vi "运维调试_采配水GD.vi"() -> ()   [LabVIEW 2016, in "PLC.lvlib"]
uses:
  PLC.lvlib
  control/switch.ctl
  <vilib>/Plasmionique/MB Master/MB_Master/MB_Master.lvclass
  <vilib>/Utility/miscctls.llb/LVPointTypeDef.ctl
  <vilib>/Plasmionique/MB Master/MB_Master_Serial/MB_Master_Serial.lvclass
  E:/Program Files (x86)/National Instruments/LabVIEW 2016/vi.lib/Plasmionique/MB Master/MB_Master/MB_Master.lvclass
  <vilib>/Plasmionique/MB Master/MB_Master_TCP/MB_Master_TCP.lvclass
  <vilib>/Plasmionique/MB Master/MB Master.lvlib
panel:
  in  "选项卡控件":enum32{"流程图", "控制面板"}(tab)
  in  "泵2进样阀":T1
  in  "泵1进样阀":T1
  in  "除藻泵阀":T2
  in  "自来水出水阀V7":T2
  in  "空压机阀":T3
  in  "增压泵M3":T4
  in  "空压机":T5
  in  "除藻泵M5":T6
  in  "泵1反冲洗阀V10":T2
  in  "泵2反冲洗阀V11":T2
  out "水流开关X2":T7
  in  "手动调节阀3":T8
  in  "采水泵M2":T9
  in  "采水泵M1":T9
  in  "氨氮水样池排液阀V15":T1
  in  "过滤反冲洗阀V14":T10
  in  "过滤进样阀V12":T11
  in  "配水泵M4":T3
  in  "过滤回流阀V13":T12
  in  "手动调节阀2":T13
  in  "压力开关":T14
  in  "手动调节阀":T8
  in  "流通池排液阀V4":T1
  in  "沉淀池排液阀V5":T1
  out "流通池液位开关X0":T15
  in  "沉淀池反冲洗阀-V9":T16
  in  "流通池反冲洗阀-V8":T16
  out "沉淀池液位开关X1":T15
  in  "M1":T17
  in  "M2":T17
  in  "V8":T17
  in  "V9":T17
  in  "V5":T17
  in  "V4":T17
  in  "V6":T17
  in  "V7":T17
  in  "V1":T17
  in  "V2":T17
  in  "V10":T17
  in  "V11":T17
  in  "M3":T17
  out "泵1进样阀计时":dbl
  out "泵2进样阀计时":dbl
  out "流通池反冲洗阀计时":dbl
  out "沉淀池反冲洗阀计时":dbl
  out "沉淀池排液阀计时":dbl
  out "流通池排液阀计时":dbl
  out "进气阀计时":dbl
  out "自来水出水阀计时":dbl
  out "泵1反冲洗阀计时":dbl
  out "泵2反冲洗阀计时":dbl
  out "M1工作计时":dbl
  out "M2工作计时":dbl
  out "增压泵计时":dbl
  in  "V3-G":T17
  in  "V3-R":T17
  out "流通池进样阀计时":dbl
  out "沉淀池进样阀计时":dbl
  in  "V13-R":T17
  in  "V14-G":T17
  in  "V12":T17
  in  "V13-G":T17
  in  "V14-R":T17
  out "过滤进样阀计时":dbl
  out "过滤回流阀计时":dbl
  out "过滤废水阀计时":dbl
  out "过滤反冲洗阀计时":dbl
  out "过滤出水阀计时":dbl
  in  "V15":T17
  in  "M4":T17
  out "氨氮水样池排液阀计时":dbl
  out "配水泵计时":dbl
  in  "63μm反冲洗阀":T17
  out "63μm反冲洗阀计时":dbl
  in  "除藻_M5":T17
  out "除藻计时":dbl
  in  "R124":u16(ring) caption="除藻工作模式" items=["手动", "自动"]
  out "R125":i16 caption="除藻时间"
  in  "连接设置":bool
  out "供水压力":sgl format="%#.4f"
  in  "63μm反冲洗阀启用":bool caption="63μm反冲洗阀"
  out "过滤压力":sgl format="%#.4f"
  in  "三级过滤系统":bool
  out "X8":bool caption="氨氮水样池液位开关_SL3"
  out "R122":i16 caption="氨氮水样池润洗时间"
  out "R123":i16 caption="过滤装置清洗时间"
  out "R121":i16 caption="过滤装置润洗时间"
  out "R120":i16 caption="加标回收配水时间"
  out "R116":i16 caption="储水时间设定"
  out "R115":i16 caption="清洗频次设定"
  out "R114":i16 caption="排液时间"
  out "R113":i16 caption="沉淀池清洗时间"
  out "R112":i16 caption="流通池清洗时间"
  out "R111":i16 caption="吹气时间"
  out "R110":i16 caption="外部管路清洗时间"
  out "R109":i16 caption="配水时间"
  out "R108":i16 caption="沉淀时间"
  out "R107":i16 caption="液位开关报警时间"
  out "R106":i16 caption="进样超时时间"
  out "R105":i16 caption="沉淀池润洗时间"
  out "R104":i16 caption="流通池润洗时间"
  out "状态":u16[](array[numeric])
  in  "更新程序":bool
  out "清洗次数":u16
  out "当前启动泵号":enum16{"1号泵", "2号泵"}(ring)
  in  "R117":u16(ring) caption="水箱储水水体" items=["自来水", "水样"]
  out "X2":bool caption="进样水流开关_JY"
  out "采配水版本号":string
  out "通讯故障":bool
  in  "R102":u16(ring) caption="采水泵工作模式" items=["泵1单泵单管路", "泵2单泵单管路", "双泵双管路"]
  out "X7":bool caption="烟雾报警_YW"
  out "X6":bool caption="泵2过载报警_KM2"
  out "X5":bool caption="泵1过载报警_KM1"
  out "X4":bool caption="外部电源断电报警_DD1"
  out "X3":bool caption="水浸报警_SJ"
  out "X1":bool caption="沉淀池液位开关_YE2"
  out "X0":bool caption="流通池液位开关_YE1"
  out "集成报警信息":string
  out "R2":i16
  out "R1":i16
  out "多列列表框":i32(listbox)
  in  "返回":bool
  in  "参数设置":bool
  in  "单步启动":bool
  in  "启动":bool
  in  "停止":bool
  # "S"
  # "S"
  # "S"
  # "S"
  # "S"
  # "S"
  # "S"
  # "S"
  # "S"
  # "S"
  # "S"
  # "S"
  # "S"
  # "S"
  # "次"
  # "S"
  # "S"
  # "S"
  # "供水压力："
  # "Mpa"
  # "过滤压力："
  # "Mpa"
  # "单步计时："
  # "s"
  # "流程计时："
  # "s"
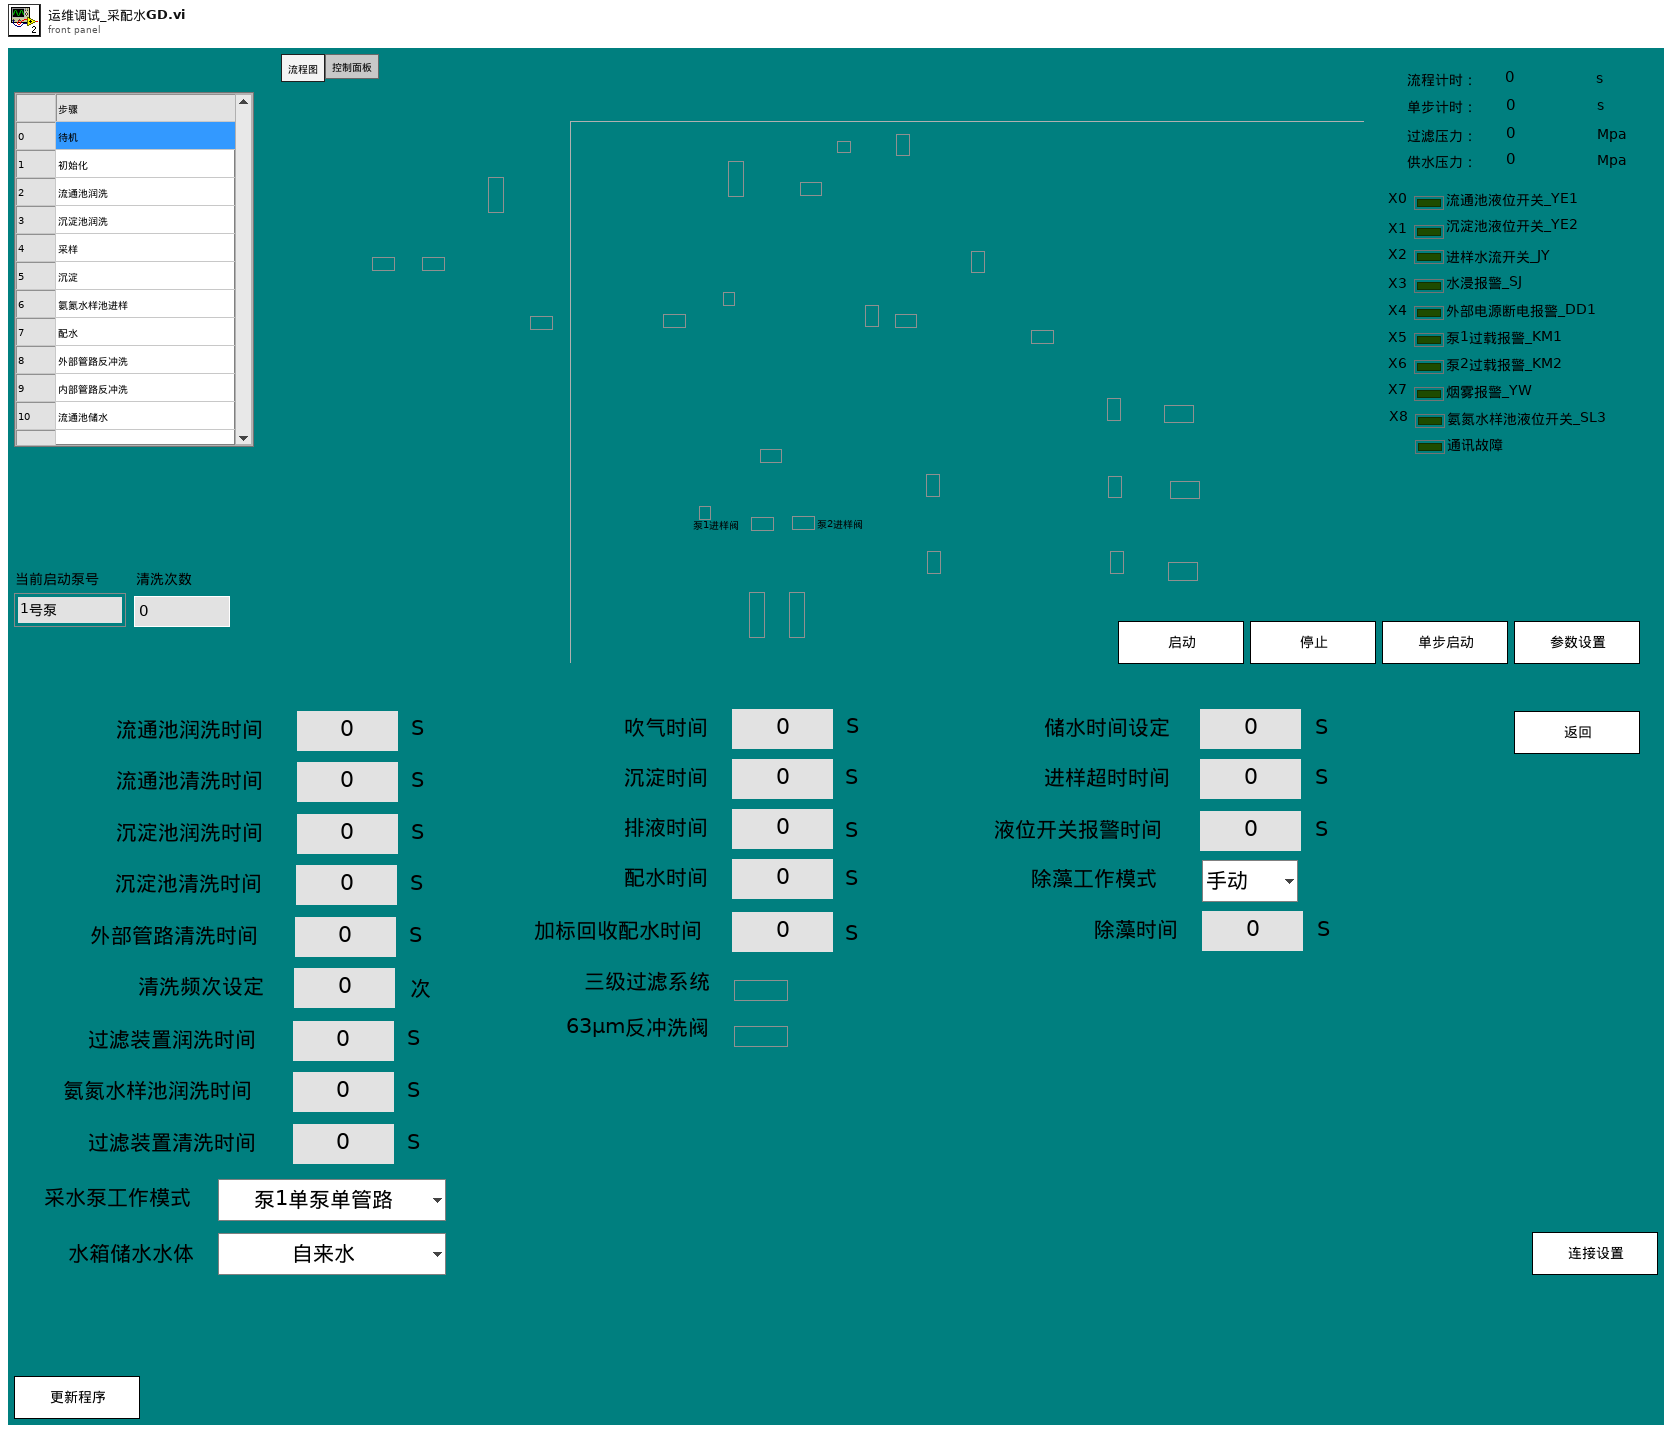
[diagram p1: front panel]
types:
  T1 = typedef "排液阀.ctl" = bool
  T2 = typedef "过滤进样阀.ctl" = bool
  T3 = typedef "电磁阀.ctl" = bool
  T4 = typedef "增压泵.ctl" = bool
  T5 = typedef "空压机.ctl" = bool
  T6 = typedef "除藻泵.ctl" = bool
  T7 = typedef "水流开关.ctl" = bool
  T8 = typedef "手动调节阀.ctl" = bool
  T9 = typedef "采水泵.ctl" = bool
  T10 = typedef "过滤出水阀.ctl" = bool
  T11 = typedef "过滤进样阀左.ctl" = bool
  T12 = typedef "三通电动球阀.ctl" = bool
  T13 = typedef "手动调节阀2.ctl" = bool
  T14 = typedef "压力开关.ctl" = bool
  T15 = typedef "浮子液位开关.ctl" = bool
  T16 = typedef "反冲洗阀.ctl" = bool
  T17 = typedef "PLC.lvlib/switch.ctl" = bool
  T18 = typedef "参数.ctl" = cluster{"测试模式":enum16{"水样测试", "平行样测试", "集成干预测试", "加标回收"}, "参数启用":T19}
  T19 = typedef "启动参数.ctl" = cluster{"氨氮":bool, "总磷":bool, "总氮":bool, "多参数":bool, "CODmn":bool, "CODCr":bool, "氟化物":bool, "超标留样":bool, "重金属":bool, "挥发酚":bool}
  T20 = cluster{"R100":i16, "R101":i16, "R102":i16, "R103":i16, "R104":i16, "R105":i16, "R106":i16, "R107":i16, "R108":i16, "R109":i16, "R110":i16, "R111":i16, "R112":i16, "R113":i16, "R114":i16, "R115":i16, "R116":i16, "R117":i16, "R118":i16, "R119":i16, "R120":i16, "R121":i16, "R122":i16, "R123":i16, "R124":i16, "R125":i16, "R126":i16, "R127":i16, "R128":i16, "R129":i16, "R130":i16, "R131":i16, "R132":i16, "R133":i16, "R134":i16, "R135":i16, "R136":i16}
  T21 = typedef "LVPointTypeDef.ctl" = cluster{"Horizontal":i16, "Vertical":i16}
  T22 = typedef "采配水类型.ctl" = enum16{"V1", "V2", "V3", "V4", "室内V1", "室内V2", "固定站V1", "固定站V2", "浮船V1", "浮船V2", "养殖渭水"}
  T23 = cluster{"R0":i16, "R1":i16, "R2":i16, "R3":i16, "R4":i16, "R5":i16, "R6":i16, "R7":i16, "R8":i16, "R9":i16, "R10":i16, "R11":i16, "R12":i16, "R13":i16, "R14":i16, "R15":i16, "R16":i16, "R17":i16, "R18":i16, "R19":i16, "R20":i16, "R21":i16, "R22":i16, "R23":i16, "R24":i16, "R25":i16, "R26":i16, "R27":i16, "R28":i16, "R29":i16, "R30":i16, "R31":i16, "R32":i16, "R33":i16, "R34":i16, "R35":i16, "R36":i16, "R37":i16, "R38":i16, "R39":i16, "R40":i16, "R41":i16, "R42":i16, "R43":i16, "R44":i16, "R45":i16, "R46":i16, "R47":i16, "R48":i16, "R49":i16, "R50":i16, "R51":i16, "R52":i16, "R53":i16, "R54":i16, "R55":i16, "R56":i16, "R57":i16, "R58":i16, "R59":i16, "R60":i16, "R61":i16, "R62":i16, "R63":i16, "R64":i16, "R65":i16, "R66":i16, "R67":i16, "R68":i16, "R69":i16, "R70":i16, "R71":i16, "R72":i16, "R73":i16, "R74":i16, "R75":i16, "R76":i16, "R77":i16, "R78":i16, "R79":i16}
  T24 = cluster{"seconds since 1Jan1904":timestamp, "table输入":string, string, "table输入":string}
  T25 = cluster{"命令":string, cluster{"starting address":u16, "holding register value":u16}}
  T26 = cluster{"命令":string, "数据":cluster{"starting address":u16, "holding register value":u16}}
  T27 = cluster{"命令":string, "数据":cluster{"starting address":u16, "holding register values":u16[]}}
  T28 = cluster{"命令":string, "data":cluster{"starting address":u16, "coil values":bool[]}}
  T29 = cluster{"测试模式":enum16{"水样测试", "平行样测试", "集成干预测试", "加标回收"}, "参数启用":T19}
  T30 = cluster{"baud rate (bps)":u32, "stop bits":u16, "parity":u16, "flow control":u16, "timeout":u32, "retries":i32}
  T31 = cluster{"starting address":u16, "holding register values":u16[]}
  T32 = cluster{"starting address":u16, "holding register value":u16}
  T33 = cluster{"starting address":u16, "coil values":bool[]}
  T34 = cluster{"连接类型":enum16{"串口", "TCP"}, "串口":string, "IP":string, "PORT":u16}
  T35 = cluster{"Registers[0]":u16, "Registers[1]":u16, "Registers[2]":u16, "Registers[3]":u16, "Registers[4]":u16, "Registers[5]":u16, "Registers[6]":u16, "Registers[7]":u16, "Registers[8]":u16, "Registers[9]":u16, "Registers[10]":u16, "Registers[11]":u16, "Registers[12]":u16, "Registers[13]":u16, "Registers[14]":u16, "Registers[15]":u16, "Registers[16]":u16, "Registers[17]":u16, "Registers[18]":u16, "Registers[19]":u16, "Registers[20]":u16, "Registers[21]":u16, "Registers[22]":u16, "Registers[23]":u16, "Registers[24]":u16, "Registers[25]":u16, "Registers[26]":u16, "Registers[27]":u16, "Registers[28]":u16, "Registers[29]":u16, "Registers[30]":u16, "Registers[31]":u16, "Registers[32]":u16, "Registers[33]":u16, "Registers[34]":u16, "Registers[35]":u16, "Registers[36]":u16, "Registers[37]":u16, "Registers[38]":u16, "Registers[39]":u16, "Registers[40]":u16, "Registers[41]":u16, "Registers[42]":u16, "Registers[43]":u16, "Registers[44]":u16, "Registers[45]":u16, "Registers[46]":u16, "Registers[47]":u16, "Registers[48]":u16, "Registers[49]":u16, "Registers[50]":u16, "Registers[51]":u16, "Registers[52]":u16, "Registers[53]":u16, "Registers[54]":u16, "Registers[55]":u16, "Registers[56]":u16, "Registers[57]":u16, "Registers[58]":u16, "Registers[59]":u16, "Registers[60]":u16, "Registers[61]":u16, "Registers[62]":u16, "Registers[63]":u16, "Registers[64]":u16, "Registers[65]":u16, "Registers[66]":u16, "Registers[67]":u16, "Registers[68]":u16, "Registers[69]":u16, "Registers[70]":u16, "Registers[71]":u16, "Registers[72]":u16, "Registers[73]":u16, "Registers[74]":u16, "Registers[75]":u16, "Registers[76]":u16, "Registers[77]":u16, "Registers[78]":u16, "Registers[79]":u16}
  T36 = cluster{"Registers[0]":u16, "Registers[1]":u16, "Registers[2]":u16, "Registers[3]":u16, "Registers[4]":u16, "Registers[5]":u16}
  T37 = cluster{"Registers[0]":u16, "Registers[1]":u16, "Registers[2]":u16, "Registers[3]":u16, "Registers[4]":u16, "Registers[5]":u16, "Registers[6]":u16, "Registers[7]":u16, "Registers[8]":u16, "Registers[9]":u16, "Registers[10]":u16, "Registers[11]":u16, "Registers[12]":u16, "Registers[13]":u16, "Registers[14]":u16, "Registers[15]":u16, "Registers[16]":u16, "Registers[17]":u16, "Registers[18]":u16, "Registers[19]":u16, "Registers[20]":u16, "Registers[21]":u16, "Registers[22]":u16, "Registers[23]":u16, "Registers[24]":u16, "Registers[25]":u16, "Registers[26]":u16, "Registers[27]":u16, "Registers[28]":u16, "Registers[29]":u16, "Registers[30]":u16, "Registers[31]":u16, "Registers[32]":u16, "Registers[33]":u16, "Registers[34]":u16, "Registers[35]":u16, "Registers[36]":u16}
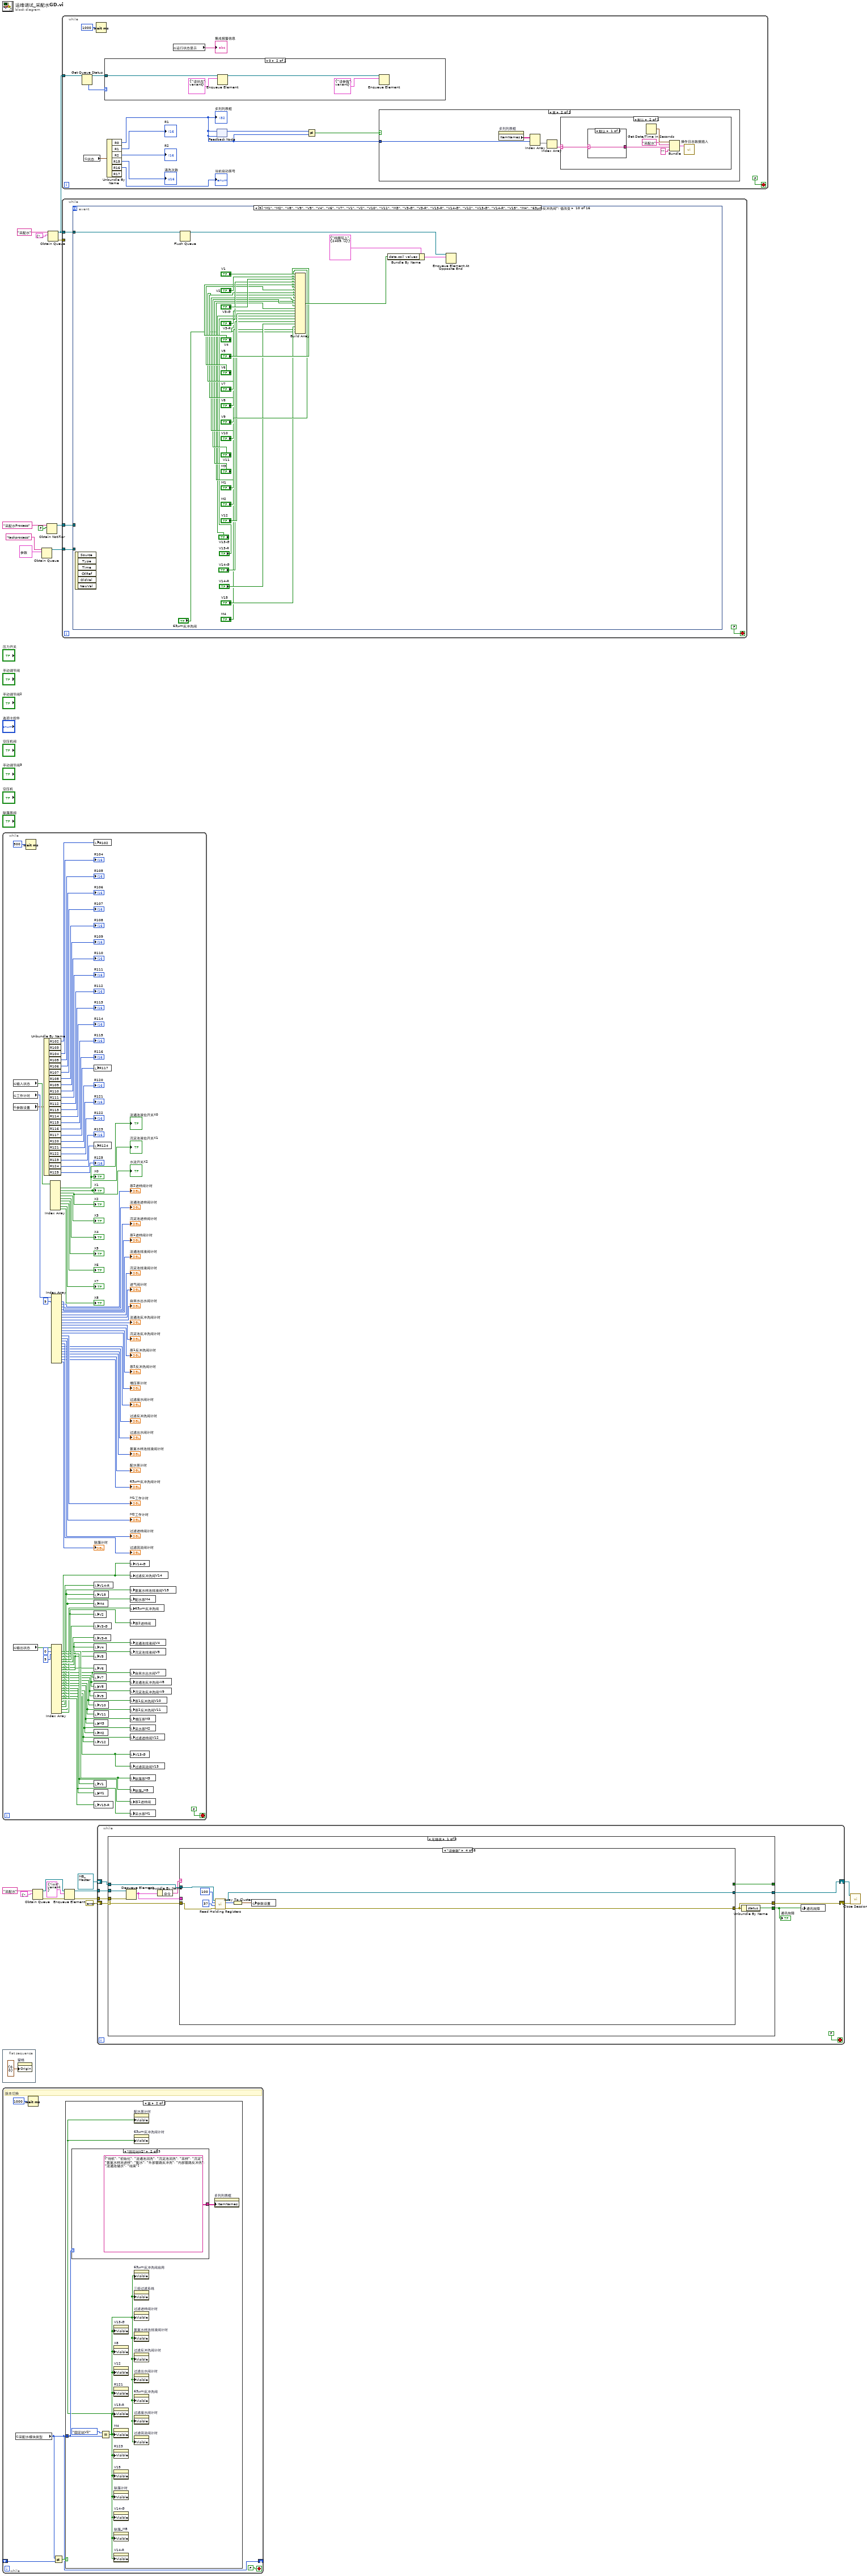
[diagram p0: block diagram]
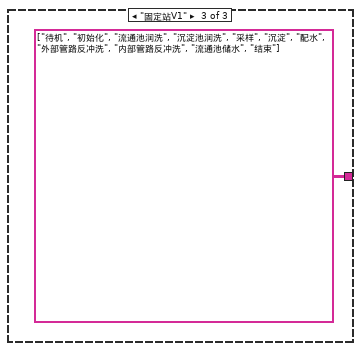
[diagram p4: hidden frame]
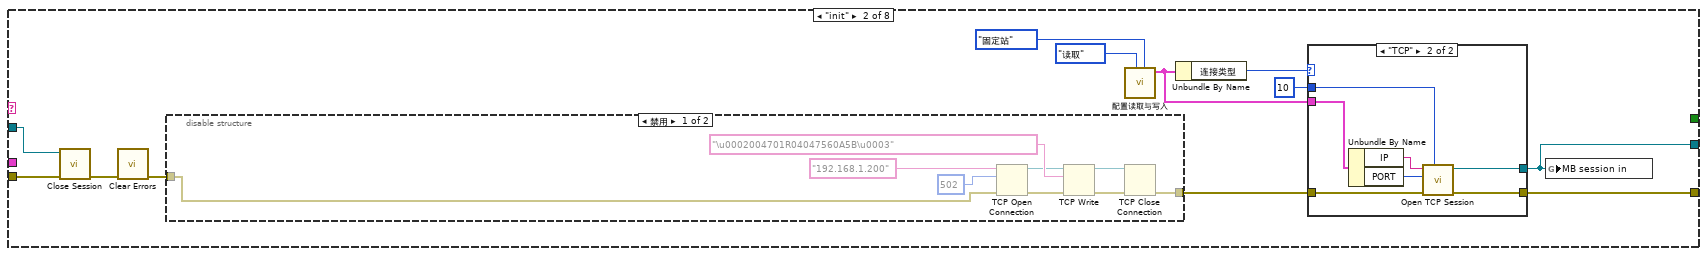
[diagram p6: hidden frame]
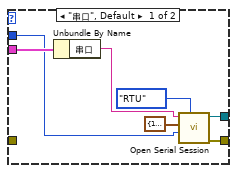
[diagram p7: hidden frame]
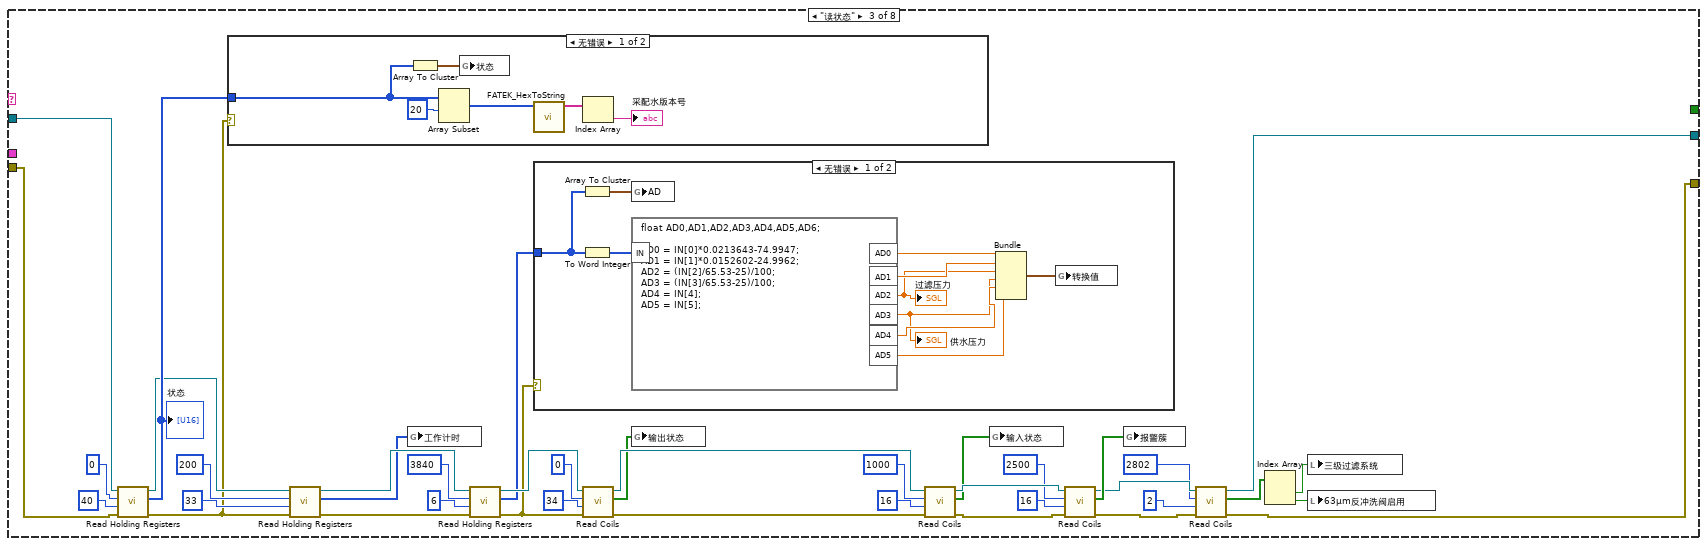
[diagram p9: hidden frame]
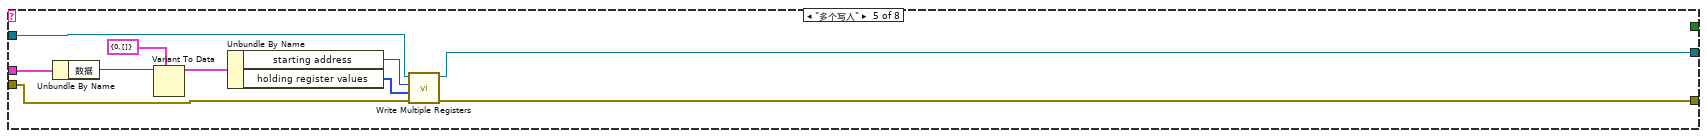
[diagram p12: hidden frame]
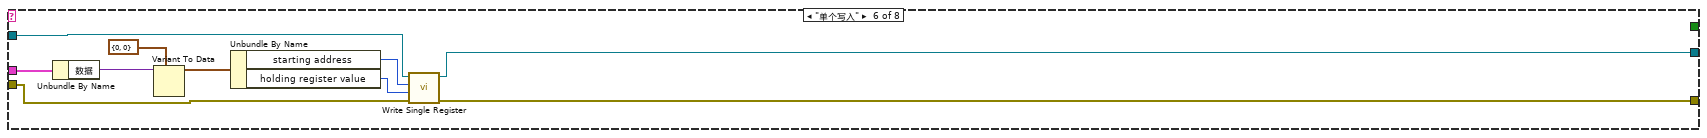
[diagram p13: hidden frame]
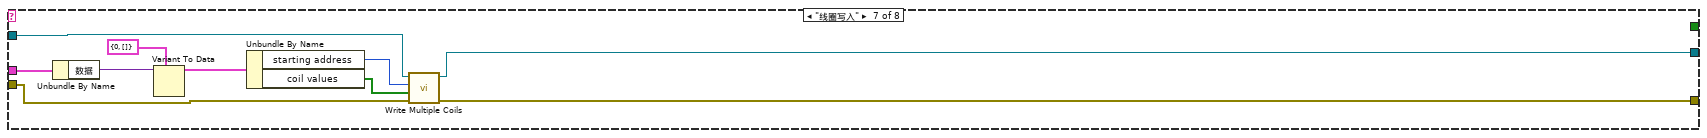
[diagram p14: hidden frame]
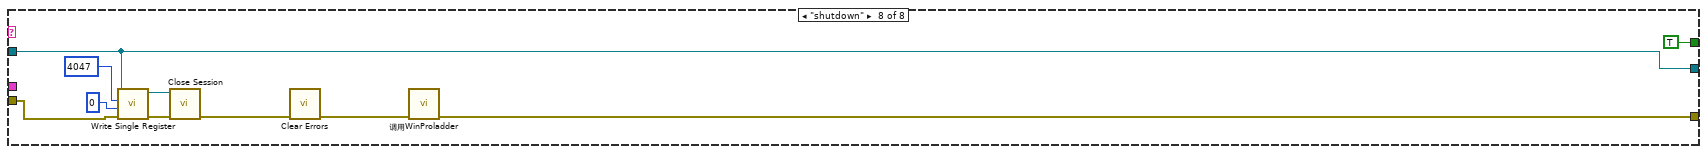
[diagram p15: hidden frame]
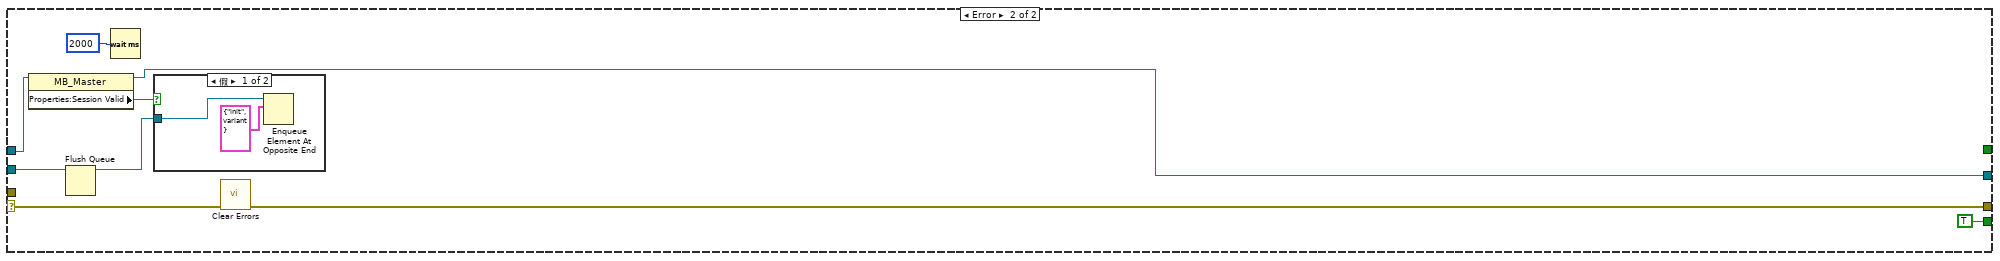
[diagram p16: hidden frame]
diagram:
  n1 = while {
    stop <- FALSE stop-if-true
    n2 = global read "采配水全局变量.vi" "输入状态"() -> (w101:bool[])
    n3 = global read "采配水全局变量.vi" "工作计时"() -> (w95:u16[])
    n4 = global read "采配水全局变量.vi" "参数设置"() -> (w93:T20)
    n5 = global read "采配水全局变量.vi" "输出状态"() -> (w107:bool[])
    n6 = Wait (ms)(milliseconds to wait=u32 500 ("等待时间（毫秒）")) -> ()  [unwired: 1 out]
    n7 = Unbundle By Name(w93) -> ("R102"=w92:i16, "R104"=→"R104":i16, "R105"=→"R105":i16, "R106"=→"R106":i16, "R107"=→"R107":i16, "R108"=→"R108":i16, "R109"=→"R109":i16, "R110"=→"R110":i16, "R111"=→"R111":i16, "R112"=→"R112":i16, "R113"=→"R113":i16, "R114"=→"R114":i16, "R115"=→"R115":i16, "R116"=→"R116":i16, "R117"=w78:i16, "R120"=→"R120":i16, "R121"=→"R121":i16, "R122"=→"R122":i16, "R123"=→"R123":i16, "R124"=w45:i16, "R125"=→"R125":i16)  [unwired: 1 out]
    n8 = Index Array(array=w101) -> (element #1=→"X0" →"流通池液位开关X0":bool, element #2=→"X1" →"沉淀池液位开关X1":bool, element #3=→"X2" →"水流开关X2":bool, element #4=→"X3":bool, element #5=→"X4":bool, element #6=→"X5":bool, element #7=→"X6":bool, element #8=→"X7":bool, element #9=→"X8":bool)  [unwired: 9 in]
    n9 = Index Array(array=w95, index #1=9 ("索引")) -> (element #1=→"泵1进样阀计时":u16, element #2=→"泵2进样阀计时":u16, element #3=→"流通池进样阀计时":u16, element #4=→"沉淀池进样阀计时":u16, element #5=→"流通池排液阀计时":u16, element #6=→"沉淀池排液阀计时":u16, element #7=→"进气阀计时":u16, element #8=→"自来水出水阀计时":u16, element #9=→"流通池反冲洗阀计时":u16, element #10=→"沉淀池反冲洗阀计时":u16, element #11=→"泵1反冲洗阀计时":u16, element #12=→"泵2反冲洗阀计时":u16, element #13=→"增压泵计时":u16, element #14=→"M1工作计时":u16, element #15=→"M2工作计时":u16, element #16=→"过滤进样阀计时":u16, element #17=→"过滤回流阀计时":u16, element #18=→"过滤废水阀计时":u16, element #19=→"过滤反冲洗阀计时":u16, element #20=→"过滤出水阀计时":u16, element #21=→"氨氮水样池排液阀计时":u16, element #22=→"配水泵计时":u16, element #23=→"63μm反冲洗阀计时":u16, element #24=→"除藻计时":u16)  [unwired: 23 in]
    n10 = Index Array(array=w107, index #1=0 ("索引"), index #2=9 ("索引")) -> (element #1=w39:bool, element #2=w38:bool, element #3=w37:bool, element #4=w105:bool, element #5=w104:bool, element #6=w36:bool, element #7=w35:bool, element #8=w103:bool, element #9=w34:bool, element #10=w33:bool, element #11=w32:bool, element #12=w31:bool, element #13=w30:bool, element #14=w29:bool, element #15=w28:bool, element #16=w27:bool, element #17=w26:bool, element #18=w25:bool, element #19=w74:bool, element #20=w24:bool, element #21=w73:bool, element #22=w23:bool, element #23=w22:bool, element #24=w70:bool)  [unwired: 22 in]
    n11 = local write "R102"(w92) -> ()
    n12 = local write "R117"(w78) -> ()
    n13 = local write "R124"(w45) -> ()
    n14 = local write "V14-R"(w73) -> ()
    n15 = local write "V15"(w23) -> ()
    n16 = local write "M4"(w22) -> ()
    n17 = local write "V2"(w37) -> ()
    n18 = local write "V3-G"(w105) -> ()
    n19 = local write "V3-R"(w104) -> ()
    n20 = local write "V4"(w36) -> ()
    n21 = local write "V5"(w35) -> ()
    n22 = local write "V6"(w103) -> ()
    n23 = local write "V7"(w34) -> ()
    n24 = local write "V8"(w33) -> ()
    n25 = local write "V9"(w32) -> ()
    n26 = local write "V10"(w31) -> ()
    n27 = local write "V11"(w30) -> ()
    n28 = local write "M3"(w29) -> ()
    n29 = local write "M2"(w27) -> ()
    n30 = local write "V12"(w26) -> ()
    n31 = local write "V1"(w38) -> ()
    n32 = local write "M1"(w28) -> ()
    n33 = local write "V13-R"(w74) -> ()
    n34 = local write "V14-G"(w24) -> ()
    n35 = local write "过滤反冲洗阀V14"(w24) -> ()
    n36 = local write "氨氮水样池排液阀V15"(w23) -> ()
    n37 = local write "配水泵M4"(w22) -> ()
    n38 = local write "63μm反冲洗阀"(w70) -> ()
    n39 = local write "泵2进样阀"(w37) -> ()
    n40 = local write "流通池排液阀V4"(w36) -> ()
    n41 = local write "沉淀池排液阀V5"(w35) -> ()
    n42 = local write "自来水出水阀V7"(w34) -> ()
    n43 = local write "流通池反冲洗阀-V8"(w33) -> ()
    n44 = local write "沉淀池反冲洗阀-V9"(w32) -> ()
    n45 = local write "泵1反冲洗阀V10"(w31) -> ()
    n46 = local write "泵2反冲洗阀V11"(w30) -> ()
    n47 = local write "增压泵M3"(w29) -> ()
    n48 = local write "采水泵M2"(w27) -> ()
    n49 = local write "过滤进样阀V12"(w26) -> ()
    n50 = local write "V13-G"(w25) -> ()
    n51 = local write "过滤回流阀V13"(w25) -> ()
    n52 = local write "除藻泵M5"(w39) -> ()
    n53 = local write "除藻_M5"(w39) -> ()
    n54 = local write "泵1进样阀"(w38) -> ()
    n55 = local write "采水泵M1"(w28) -> ()
  }
  n56 = flat-sequence {
    frame #0 {
      n57 = property on="窗格" class="Pane"("Origin"=T21 {"Horizontal"=0, "Vertical"=0} ("原点")) -> ()  [unwired: 2 in, 2 out]
    }
  }
  n58 = while {
    shift-right: [w110] -> _
    shift-left: _ -> [w113]
    stop <- FALSE stop-if-true
    # "版本切换"
    n59 = global read "系统设置全局变量.vi" "采配水模块类型"() -> (w110:T22)
    n60 = Wait (ms)(milliseconds to wait=u32 1000 ("等待时间（毫秒）")) -> ()  [unwired: 1 out]
    n61 = Not Equal?(x=w110, y=w113) -> (x != y?=w111:bool)
    n62 = case shown="真" w111 {
      tunnel: w110 -> [_ w117]
      frame False {
      }
      frame True {
        n63 = case shown="\"固定站V2\"" w117 {
          tunnel: [_ string[][] [["待机"], ["初始化"], ["流通池润洗"], ["沉淀池润洗"], ["采样"], ["沉淀"], ["氨氮水样池进样"], ["配水"], ["外部管路反冲洗"], ["内部管路反冲洗"], ["流通池储水"], ["结束"]] ("项名") string[][] [["待机"], ["初始化"], ["流通池润洗"], ["沉淀池润洗"], ["采样"], ["沉淀"], ["配水"], ["外部管路反冲洗"], ["内部管路反冲洗"], ["流通池储水"], ["结束"]] ("项名")] -> w116
          frame Default {
          }
          frame "固定站V2" {
          }
          frame "固定站V1" {
          }
        }
        n64 = Equal?(x=采配水类型."固定站V2", y=w117) -> (x = y?=w115:bool)
        n65 = property on="V13-G" class="Bool (严格)"("Visible"=w115) -> ()  [unwired: 2 in, 2 out]
        n66 = property on="X8" class="Bool (严格)"("Visible"=w115) -> ()  [unwired: 2 in, 2 out]
        n67 = property on="V12" class="Bool (严格)"("Visible"=w115) -> ()  [unwired: 2 in, 2 out]
        n68 = property on="R121" class="DigNum (严格)"("Visible"=w115) -> ()  [unwired: 2 in, 2 out]
        n69 = property on="V13-R" class="Bool (严格)"("Visible"=w115) -> ()  [unwired: 2 in, 2 out]
        n70 = property on="M4" class="Bool (严格)"("Visible"=w115) -> ()  [unwired: 2 in, 2 out]
        n71 = property on="R123" class="DigNum (严格)"("Visible"=w115) -> ()  [unwired: 2 in, 2 out]
        n72 = property on="V15" class="Bool (严格)"("Visible"=w115) -> ()  [unwired: 2 in, 2 out]
        n73 = property on="除藻计时" class="DigNum (严格)"("Visible"=w115) -> ()  [unwired: 2 in, 2 out]
        n74 = property on="V14-G" class="Bool (严格)"("Visible"=w115) -> ()  [unwired: 2 in, 2 out]
        n75 = property on="除藻_M5" class="Bool (严格)"("Visible"=w115) -> ()  [unwired: 2 in, 2 out]
        n76 = property on="V14-R" class="Bool (严格)"("Visible"=w115) -> ()  [unwired: 2 in, 2 out]
        n77 = property on="配水泵计时" class="DigNum (严格)"("Visible"=w115) -> ()  [unwired: 2 in, 2 out]
        n78 = property on="63μm反冲洗阀计时" class="DigNum (严格)"("Visible"=w115) -> ()  [unwired: 2 in, 2 out]
        n79 = property on="63μm反冲洗阀启用" class="Bool (严格)"("Visible"=w115) -> ()  [unwired: 2 in, 2 out]
        n80 = property on="三级过滤系统" class="Bool (严格)"("Visible"=w115) -> ()  [unwired: 2 in, 2 out]
        n81 = property on="过滤进样阀计时" class="DigNum (严格)"("Visible"=w115) -> ()  [unwired: 2 in, 2 out]
        n82 = property on="氨氮水样池排液阀计时" class="DigNum (严格)"("Visible"=w115) -> ()  [unwired: 2 in, 2 out]
        n83 = property on="过滤反冲洗阀计时" class="DigNum (严格)"("Visible"=w115) -> ()  [unwired: 2 in, 2 out]
        n84 = property on="过滤出水阀计时" class="DigNum (严格)"("Visible"=w115) -> ()  [unwired: 2 in, 2 out]
        n85 = property on="63μm反冲洗阀" class="Bool (严格)"("Visible"=w115) -> ()  [unwired: 2 in, 2 out]
        n86 = property on="过滤废水阀计时" class="DigNum (严格)"("Visible"=w115) -> ()  [unwired: 2 in, 2 out]
        n87 = property on="过滤回流阀计时" class="DigNum (严格)"("Visible"=w115) -> ()  [unwired: 2 in, 2 out]
        n88 = property on="多列列表框" class="MCListbox (严格)"("ItemNames"=w116) -> ()  [unwired: 2 in, 2 out]
      }
    }
  }
  n89 = Obtain Queue(name (unnamed)="采配水" ("名称（未命名）"), element data type=cluster{"命令":string, "数据":variant} {"命令"="", "数据"=variant}) -> (queue out=w12:refnum<queue>, error out=w11:errorcluster)  [unwired: 3 in, 1 out]
  n90 = Obtain Queue(name (unnamed)="taskprocess" ("名称（未命名）"), element data type=T18 {"测试模式"=enum."水样测试", "参数启用"={"氨氮"=FALSE, "总磷"=FALSE, "总氮"=FALSE, "多参数"=FALSE, "CODmn"=FALSE, "CODCr"=FALSE, "氟化物"=FALSE, "超标留样"=FALSE, "重金属"=FALSE, "挥发酚"=FALSE}} ("参数")) -> (queue out=w2:refnum<queue>)  [unwired: 3 in, 2 out]
  n91 = Obtain Notifier(name (unnamed)="采配水Process" ("名称（未命名）"), notification data type=FALSE) -> (notifier out=w15:refnum<notifier>)  [unwired: 2 in, 2 out]
  n92 = Obtain Queue(name (unnamed)="采配水" ("名称（未命名）"), element data type=cluster{"命令":string, "数据":variant} {"命令"="", "数据"=variant}) -> (queue out=w18:refnum<queue>, error out=w19:errorcluster)  [unwired: 3 in, 1 out]
  n93 = while {
    tunnel: w18 -> [w133]
    stop <- FALSE stop-if-true
    n94 = Get Queue Status(queue=w133) -> (queue out=w122:refnum<queue>, # elements in queue=w121:i32)  [unwired: 2 in, 6 out]
    n95 = global read "采配水全局变量.vi" "状态"() -> (w132:T23)
    n96 = Wait (ms)(milliseconds to wait=u32 1000 ("等待时间（毫秒）")) -> ()  [unwired: 1 out]
    n97 = case shown="0" w121 {
      tunnel: w122 -> [_ w135]
      frame Default {
      }
      frame 0 {
        n98 = Enqueue Element(queue=w135, element=cluster{"命令":string, "数据":variant} {"命令"="读状态", "数据"=variant} ("元素")) -> (queue out=w136:refnum<queue>)  [unwired: 2 in, 2 out]
        n99 = Enqueue Element(queue=w136, element=cluster{"命令":string, "数据":variant} {"命令"="读参数", "数据"=variant} ("元素")) -> ()  [unwired: 2 in, 3 out]
      }
    }
    n100 = Unbundle By Name(w132) -> ("R0"=w125:i16, "R1"=→"R1":i16, "R2"=→"R2":i16, "R15"=→"清洗次数":i16, "R16"=→"当前启动泵号":i16)  [unwired: 1 out]
    "多列列表框" <- w125
    n101 = global read "采配水全局变量.vi" "运行状态显示"() -> (→"集成报警信息":string)
    n102 = feedback-in #1(w125) -> ()
    n103 = feedback #1(w125) -> (w126:i16)
    n104 = Not Equal?(x=w126, y=w125) -> (x != y?=w129:bool)
    n105 = case shown="真" w129 {
      tunnel: w125 -> [_ w141]
      frame False {
      }
      frame True {
        n106 = property on="多列列表框" class="MCListbox (严格)"() -> ("ItemNames"=w142:string[][])  [unwired: 2 in, 2 out]
        n107 = Index Array(array=w142, index (row)=w141) -> (element=w140:string[])  [unwired: 1 in]
        n108 = Index Array(array=w140) -> (element=w139:string)  [unwired: 1 in]
        n109 = case shown="默认" w139 {
          selector: w139 -> [_ w145]
          frame "待机" {
          }
          frame Default {
            n110 = case shown="默认" w145 {
              selector: w145 -> [w149 _ _]
              tunnel: [w149 "<<启动" "结束>>"] -> w144
              frame Default {
              }
              frame "初始化" {
              }
              frame "结束" {
              }
            }
            n111 = Get Date/Time In Seconds() -> (seconds since 1Jan1904=w148:timestamp)
            n112 = Bundle("seconds since 1Jan1904"=w148, "table输入"="采配水", w144, "table输入"="") -> (w143:T24)  [unwired: 1 in]
            n113 = call "操作日志数据插入.vi"("data"=w143) -> ()  [unwired: 9 in, 1 out]
          }
        }
      }
    }
  }
  n114 = while {
    tunnel: w18 -> [w154]
    tunnel: w19 -> [_]
    tunnel: w15 -> [w153]
    tunnel: w2 -> [w152]
    stop <- FALSE stop-if-true
    n115 = event shown="[9] \"M1\", \"M2\", \"V8\", \"V9\", \"V5\", \"V4\", \"V6\", \"V7\", \"V1\", \"V2\", \"V10\", \"V11\", \"M3\", \"V3-G\", \"V3-R\", \"V13-R\", \"V14-G\", \"V12\", \"V13-G\", \"V14-R\", \"V15\", \"M4\", \"63μm反冲洗阀\": 值改变" {
      selector: _ -> [_ _ _ _ _ _ _ _ _ _ _ _ _ _ _ _]
      dyn-events: _ -> [_ _ _ _ _ _ _ _ _ _ _ _ _ _ _ _]
      timeout: _ -> [_ _ _ _ _ _ _ _ _ _ _ _ _ _ _ _]
      tunnel: w154 -> [_ w158 w164 _ w186 w194 _ _ _ w251 w274 w282 w290 w297 w303 w310]
      tunnel: w153 -> [_ _ w163 w168 _ _ _ _ _ _ _ _ _ _ _ _]
      tunnel: w152 -> [_ _ w161 w166 _ _ _ _ _ _ _ _ _ _ _ _]
      event Timeout {
        n116 = event-data() -> ()  [unwired: 1 in, 3 out]
      }
      event "连接设置": Value Change {
        n117 = event-data() -> ()  [unwired: 1 in, 6 out]
        n118 = call "连接配置对话框.vi"("类别"=enum16{"微站", "固定站"}."固定站") -> ("check？"=w157:bool)  [unwired: 18 in]
        n119 = case shown="真" w157 {
          tunnel: w158 -> [_ w160]
          frame False {
          }
          frame True {
            n120 = Enqueue Element(queue=w160, element=cluster{"命令":string, "数据":variant} {"命令"="init", "数据"=variant} ("元素")) -> ()  [unwired: 2 in, 3 out]
          }
        }
      }
      event "停止": Value Change {
        n121 = event-data() -> ()  [unwired: 1 in, 6 out]
        n122 = Flush Queue(queue=w161) -> ()  [unwired: 1 in, 3 out]
        n123 = Send Notification(notification=TRUE ("通知"), notifier=w163) -> ()  [unwired: 1 in, 2 out]
        n124 = Enqueue Element At Opposite End(queue=w164, element=T25 {"命令"="单个写入", {"starting address"=300, "holding register value"=2}} ("元素")) -> ()  [unwired: 2 in, 3 out]
      }
      event "启动": Value Change {
        n125 = event-data() -> ()  [unwired: 1 in, 6 out]
        n126 = flat-sequence {
          tunnel: w168 -> [w170]
          tunnel: [w169] -> w167
          tunnel: w166 -> [w169]
          tunnel: w167 -> [w173]
          frame #0 {
            n127 = Cancel Notification(0:w170) -> ()  [unwired: 1 in, 3 out]
          }
          frame #1 {
            n128 = call "手动启动选择对话框.vi"() -> ("确定"=w171:bool, "输出簇"=w172:cluster{"参数启用":T19})  [unwired: 10 in]
            n129 = case shown="真" w171 {
              tunnel: w172 -> [_ w176]
              tunnel: w173 -> [_ w175]
              frame False {
              }
              frame True {
                n130 = global read "采配水全局变量.vi" "流程运行中"() -> (w174:bool)
                n131 = case shown="假" w174 {
                  tunnel: w176 -> [w179 _]
                  tunnel: w175 -> [w181 _]
                  frame False {
                    n132 = Unbundle By Name(w179) -> ("参数启用"=w178:T19)
                    n133 = Bundle("测试模式"=enum16{"水样测试", "平行样测试", "集成干预测试", "加标回收"}."水样测试", "参数启用"=w178) -> (w177:T29)  [unwired: 1 in]
                    n134 = Enqueue Element(queue=w181, element=w177) -> ()  [unwired: 2 in, 3 out]
                  }
                  frame True {
                    n135 = One Button Dialog(message="流程已启动，无需重复启动！" ("消息")) -> ()  [unwired: 1 in, 1 out]
                  }
                }
              }
            }
          }
        }
      }
      event "单步启动": Value Change {
        n136 = event-data() -> ()  [unwired: 1 in, 6 out]
        n137 = call "单步启动对话框.vi"() -> ("单步启动步骤输出"=w183:u16)  [unwired: 11 in]
        n138 = Bundle By Name(cluster=T26 {"命令"="单个写入", "数据"={"starting address"=301, "holding register value"=0}} ("元素"), "数据.holding register value"=w183) -> (w184:T26)
        n139 = Enqueue Element At Opposite End(queue=w186, element=w184) -> ()  [unwired: 2 in, 3 out]
      }
      event "R104", "R117", "R105", "R106", "R107", "R108", "R109", "R110", "R111", "R112", "R113", "R114", "R115", "R116", "R102", "R120", "R121", "R123", "R122": Value Change {
        n140 = event-data() -> ()  [unwired: 1 in, 6 out]
        n141 = local read "R104"() -> (w212:i16)
        n142 = local read "R105"() -> (w211:i16)
        n143 = local read "R106"() -> (w210:i16)
        n144 = local read "R107"() -> (w209:i16)
        n145 = local read "R108"() -> (w208:i16)
        n146 = local read "R109"() -> (w207:i16)
        n147 = local read "R110"() -> (w206:i16)
        n148 = local read "R111"() -> (w205:i16)
        n149 = local read "R112"() -> (w204:i16)
        n150 = local read "R113"() -> (w203:i16)
        n151 = local read "R114"() -> (w202:i16)
        n152 = local read "R115"() -> (w201:i16)
        n153 = local read "R116"() -> (w200:i16)
        n154 = Build Array("R102", u16 0 ("元素"), w212, w211, w210, w209, w208, w207, w206, w205, w204, w203, w202, w201, w200, "R117") -> (w213:u16[])
        n155 = local read "R120"() -> (w192:i16)
        n156 = local read "R121"() -> (w190:i16)
        n157 = local read "R122"() -> (w189:i16)
        n158 = local read "R123"() -> (w188:i16)
        n159 = Build Array(w192, w190, w189, w188) -> (w191:i16[])
        n160 = Bundle By Name(cluster=T27 {"命令"="多个写入", "数据"={"starting address"=0, "holding register values"=[]}} ("元素"), "数据.starting address"=u16 102, "数据.holding register values"=w213) -> (w215:T27)
        n161 = Flush Queue(queue=w194) -> (queue out=w187:refnum<queue>)  [unwired: 1 in, 2 out]
        n162 = Bundle By Name(cluster=T27 {"命令"="多个写入", "数据"={"starting address"=0, "holding register values"=[]}} ("元素"), "数据.starting address"=u16 120, "数据.holding register values"=w191) -> (w197:T27)
        n163 = Enqueue Element At Opposite End(queue=w187, element=w215) -> (error out=w193:errorcluster)  [unwired: 2 in, 2 out]
        n164 = Enqueue Element At Opposite End(queue=w187, element=w197, error in (no error)=w193) -> ()  [unwired: 1 in, 3 out]
      }
      event "R104", "R105", "R106", "R107", "R108", "R109", "R110", "R111", "R112", "R113", "R114", "R115", "R116", "R120", "R122", "R123", "R121", "R125": Mouse Down {
        n165 = event-data() -> ("CtlRef"=w221:refnum<vi>)  [unwired: 1 in, 7 out]
        n166 = property class="DigNum (严格)"(reference=w221) -> (reference out=w219:refnum<vi>, "Value"=w220:i16)  [unwired: 1 in, 1 out]
        n167 = call "数字键盘.vi"("OldNumber"=w220) -> ("NewNumber"=w218:sgl)
        n168 = property class="DigNum (严格)"(reference=w219, "Val(Sgnl)"=w218) -> ()  [unwired: 1 in, 2 out]
      }
      event "参数设置": Value Change {
        n169 = event-data() -> ()  [unwired: 1 in, 6 out]
        n170 = property on="窗格" class="Pane"("Origin"=T21 {"Horizontal"=0, "Vertical"=628} ("原点")) -> ()  [unwired: 2 in, 2 out]
      }
      event "返回": Value Change {
        n171 = event-data() -> ()  [unwired: 1 in, 6 out]
        n172 = property on="窗格" class="Pane"("Origin"=T21 {"Horizontal"=0, "Vertical"=0} ("原点")) -> ()  [unwired: 2 in, 2 out]
      }
      event Value Change {
        n173 = event-data() -> ()  [unwired: 1 in, 6 out]
        n174 = Flush Queue(queue=w251) -> (queue out=w225:refnum<queue>)  [unwired: 1 in, 2 out]
        n175 = Build Array("V1", "V2", "V3-G", "V3-R", "V4", "V5", "V6", "V7", "V8", "V9", "V10", "V11", "M3", "M1", "M2", "V12", "V13-G", "V13-R", "V14-G", "V14-R", "V15", "M4", "63μm反冲洗阀") -> (w248:T17[])
        n176 = Bundle By Name(cluster=T28 {"命令"="线圈写入", "data"={"starting address"=2409, "coil values"=[]}} ("元素"), "data.coil values"=w248) -> (w249:T28)
        n177 = Enqueue Element At Opposite End(queue=w225, element=w249) -> ()  [unwired: 2 in, 3 out]
      }
      event Value Change {
        n178 = event-data() -> ()  [unwired: 1 in, 6 out]
        n179 = Or(x="泵1进样阀", y="泵2进样阀") -> (x .or. y?=w271:T1)
        n180 = Build Array("泵1进样阀", "泵2进样阀", w271, w271, "流通池排液阀V4", "沉淀池排液阀V5", T1 FALSE ("元素"), "自来水出水阀V7", "流通池反冲洗阀-V8", "沉淀池反冲洗阀-V9", "泵1反冲洗阀V10", "泵2反冲洗阀V11", "增压泵M3", "采水泵M1", "采水泵M2", "过滤进样阀V12", "过滤回流阀V13", T12 FALSE ("元素"), "过滤反冲洗阀V14", T10 FALSE ("元素"), "氨氮水样池排液阀V15", "配水泵M4") -> (w266:T3[])
        n181 = Bundle By Name(cluster=T28 {"命令"="线圈写入", "data"={"starting address"=2409, "coil values"=[]}} ("元素"), "data.coil values"=w266) -> (w276:T28)
        n182 = Flush Queue(queue=w274) -> (queue out=w275:refnum<queue>)  [unwired: 1 in, 2 out]
        n183 = Enqueue Element At Opposite End(queue=w275, element=w276) -> ()  [unwired: 2 in, 3 out]
      }
      event Value Change {
        n184 = event-data() -> ("CtlRef"=w279:refnum<vi>)  [unwired: 1 in, 5 out]
        n185 = property class="Bool (严格)"(reference=w279) -> ("Label.Text"=w278:string)  [unwired: 1 in, 2 out]
        n186 = case shown="\"除藻泵M5\", 默认" w278 {
          tunnel: ["除藻泵M5" "除藻_M5"] -> w281
          frame "除藻泵M5", Default {
          }
          frame "除藻_M5" {
          }
        }
        n187 = Flush Queue(queue=w282) -> (queue out=w283:refnum<queue>)  [unwired: 1 in, 2 out]
        n188 = Build Array(w281) -> (w280:T17[])
        n189 = Bundle By Name(cluster=T28 {"命令"="线圈写入", "data"={"starting address"=2432, "coil values"=[]}} ("元素"), "data.coil values"=w280) -> (w284:T28)
        n190 = Enqueue Element At Opposite End(queue=w283, element=w284) -> ()  [unwired: 2 in, 3 out]
      }
      event "R125", "R124": Value Change {
        n191 = event-data() -> ()  [unwired: 1 in, 6 out]
        n192 = local read "R125"() -> (w288:i16)
        n193 = Build Array("R124", w288) -> (w291:u16[])
        n194 = Bundle By Name(cluster=T27 {"命令"="多个写入", "数据"={"starting address"=0, "holding register values"=[]}} ("元素"), "数据.starting address"=u16 124, "数据.holding register values"=w291) -> (w292:T27)
        n195 = Enqueue Element At Opposite End(queue=w290, element=w292) -> ()  [unwired: 2 in, 3 out]
      }
      event "三级过滤系统": Value Change {
        n196 = event-data() -> ()  [unwired: 1 in, 6 out]
        n197 = Build Array("三级过滤系统") -> (w295:bool[])
        n198 = Bundle By Name(cluster=T28 {"命令"="线圈写入", "data"={"starting address"=2802, "coil values"=[]}} ("元素"), "data.coil values"=w295) -> (w299:T28)
        n199 = Flush Queue(queue=w297) -> (queue out=w298:refnum<queue>)  [unwired: 1 in, 2 out]
        n200 = Enqueue Element At Opposite End(queue=w298, element=w299) -> ()  [unwired: 2 in, 3 out]
      }
      event "63μm反冲洗阀启用": Value Change {
        n201 = event-data() -> ()  [unwired: 1 in, 6 out]
        n202 = Flush Queue(queue=w303) -> (queue out=w304:refnum<queue>)  [unwired: 1 in, 2 out]
        n203 = Build Array("63μm反冲洗阀启用") -> (w302:bool[])
        n204 = Bundle By Name(cluster=T28 {"命令"="线圈写入", "data"={"starting address"=2803, "coil values"=[]}} ("元素"), "data.coil values"=w302) -> (w305:T28)
        n205 = Enqueue Element At Opposite End(queue=w304, element=w305) -> ()  [unwired: 2 in, 3 out]
      }
      event "更新程序": Value Change {
        n206 = event-data() -> ("NewVal"=w307:bool)  [unwired: 1 in, 5 out]
        n207 = case shown="假" w307 {
          tunnel: [cluster{"命令":string, "数据":variant} {"命令"="init", "数据"=variant} ("元素") w314] -> w309
          frame False {
          }
          frame True {
            n208 = Two Button Dialog(message="警告，非专业人士请勿进行此操作！！！\n请确认是否继续？" ("消息")) -> (T button?=w313:bool)  [unwired: 2 in]
            n209 = case shown="真" w313 {
              tunnel: [_ cluster{"命令":string, "数据":variant} {"命令"="shutdown", "数据"=variant} ("元素")] -> w314
              frame False {
                n210 = local write "更新程序"(FALSE ("释放串口")) -> ()
              }
              frame True {
              }
            }
          }
        }
        n211 = Flush Queue(queue=w310) -> (queue out=w308:refnum<queue>)  [unwired: 1 in, 2 out]
        n212 = Enqueue Element(queue=w308, element=w309) -> ()  [unwired: 2 in, 3 out]
      }
    }
  }
  n213 = Enqueue Element(queue=w12, element=cluster{"命令":string, "数据":variant} {"命令"="init", "数据"=variant} ("元素"), error in (no error)=w11) -> (queue out=w7:refnum<queue>, error out=w9:errorcluster)  [unwired: 1 in, 1 out]
  n214 = while {
    tunnel: w7 -> [w322]
    tunnel: w9 -> [w321]
    shift-right: [w324] -> w6
    shift-left: refnum<class "MB_Master.lvclass"> refnum ("MB session out") -> [w323]
    shift-right: [w319] -> w4
    shift-left: errorcluster {"status"=FALSE, "code"=0, "source"=""} ("error out") -> [w318]
    stop <- FALSE stop-if-true
    n215 = case shown="无错误" w318 {
      selector: w318 -> [w332 w479]
      tunnel: [w334 w476] -> w324
      tunnel: w323 -> [w333 w477]
      tunnel: [w326 w480] -> w319
      tunnel: w322 -> [w329 w483]
      tunnel: w321 -> [w328 _]
      tunnel: [w330 _] -> _
      tunnel: [w325 TRUE ("status")] -> w317
      frame No Error {
        n216 = Dequeue Element(queue=w329, error in (no error)=w328) -> (element=w327:cluster{"命令":string, "数据":variant})  [unwired: 1 in, 3 out]
        n217 = Unbundle By Name(w327) -> ("命令"=w331:string)
        n218 = case shown="\"读参数\"" w331 {
          tunnel: [w336 w342 w382 w429 w441 w451 w461 w472] -> w334
          tunnel: w333 -> [w336 w346 w407 w434 w444 w454 w464 w472]
          tunnel: [w335 w345 w378 w428 w442 w452 w462 w465] -> w326
          tunnel: w332 -> [w335 w348 w410 w433 w443 w453 w463 w468]
          tunnel: [_ _ _ _ _ _ _ TRUE] -> w330
          tunnel: w327 -> [_ _ _ _ w440 w450 w460 _]
          frame "idle", Default {
          }
          frame "init" {
            n219 = call-dynamic "Close Session.vi"("error in (no error)"=w348, "MB session in"=w346) -> ("error out"=w347:errorcluster)  [unwired: 9 in]
            n220 = call <vilib>:"Clear Errors.vi"("error in (no error)"=w347) -> ("error out"=w344:errorcluster)  [unwired: 5 in, 1 out]
            n221 = disable-structure shown="禁用" {
              disable-tunnel: w344 -> [w364 _]
              disable-tunnel: [w363 _] -> w343
              frame Disabled {
                n222 = TCP Open Connection(address="192.168.1.200" ("IP Address"), remote port or service name=u16 502 ("远程端口或服务名称"), error in (no error)=w364) -> (connection ID=w366:refnum<k5>, error out=w365:errorcluster)  [unwired: 2 in]
                n223 = TCP Write(connection ID=w366, data in="\u0002004701R04047560A5B\u0003" ("写入缓冲区"), error in (no error)=w365) -> (connection ID out=w367:refnum<k5>, error out=w368:errorcluster)  [unwired: 1 in, 1 out]
                n224 = TCP Close Connection(connection ID=w367, error in (no error)=w368) -> (error out=w363:errorcluster)  [unwired: 1 in, 1 out]
              }
              frame Enabled {
              }
            }
            n225 = call "配置读取与写入.vi"("类别"=enum16{"微站", "固定站"}."固定站", "功能"=enum16{"读取", "写入"}."读取") -> ("连接配置 2"=w339:T34)  [unwired: 8 in, 1 out]
            n226 = Unbundle By Name(w339) -> ("连接类型"=w340:enum16{"串口", "TCP"})
            n227 = case shown="\"TCP\"" w340 {
              tunnel: [w352 w362] -> w345
              tunnel: w343 -> [_ w361]
              tunnel: [w353 w360] -> w342
              tunnel: w339 -> [w355 w359]
              tunnel: u8 10 ("Slave ID (255)") -> [w350 w356]
              frame "串口", Default {
                n228 = Unbundle By Name(w355) -> ("串口"=w354:string)
                n229 = call <vilib>:"Open Serial Session.vi"("Mode (RTU)"=enum16{"RTU", "ASCII"}."RTU", "Slave ID"=w350, "Serial Config"=T30 {"baud rate (bps)"=115200, "stop bits"=10, "parity"=0, "flow control"=0, "timeout"=1000, "retries"=1}, "VISA Resource"=w354) -> ("Error out"=w352:errorcluster, "MB_Serial session"=w353:refnum<class "MB_Master_Serial.lvclass">)  [unwired: 6 in]
              }
              frame "TCP" {
                n230 = Unbundle By Name(w359) -> ("IP"=w358:string, "PORT"=w357:u16)
                n231 = call <vilib>:"Open TCP Session.vi"("Slave ID (255)"=w356, "error in (no error)"=w361, "Port (502)"=w357, "IP Address"=w358) -> ("error out"=w362:errorcluster, "MB_TCP session"=w360:refnum<class "MB_Master_TCP.lvclass">)  [unwired: 6 in]
              }
            }
            n232 = global write "采配水全局变量.vi" "MB session in"(w342) -> ()
          }
          frame "读状态" {
            n233 = call <vilib>:"Read Holding Registers.vi"("error in (no error)"=w410, "quantity"=u16 40 ("number of holding registers"), "starting address"=u16 0, "MB session in"=w407) -> ("error out"=w375:errorcluster, "Registers"=w389:u16[], "MB session out"=w388:refnum<class "MB_Master.lvclass">)  [unwired: 5 in]
            "状态" <- w389
            n234 = case shown="无错误" w375 {
              tunnel: w389 -> [w422 _]
              frame No Error {
                n235 = Array To Cluster(array=w422) -> (cluster=w421:T35)
                n236 = Array Subset(array=w422, index=20 ("索引")) -> (w425:u16[])  [unwired: 1 in]
                n237 = global write "采配水全局变量.vi" "状态"(w421) -> ()
                n238 = call "FATEK_HexToString.vi"("数组"=w425) -> ("STRING"=w424:string[])  [unwired: 10 in]
                n239 = Index Array(array=w424) -> (element=→"采配水版本号":string)  [unwired: 1 in]
              }
              frame Error {
              }
            }
            n240 = call <vilib>:"Read Holding Registers.vi"("error in (no error)"=w375, "quantity"=u16 33, "starting address"=u16 200, "MB session in"=w388) -> ("error out"=w387:errorcluster, "Registers"=w372:u16[], "MB session out"=w386:refnum<class "MB_Master.lvclass">)  [unwired: 5 in]
            n241 = global write "采配水全局变量.vi" "工作计时"(w372) -> ()
            n242 = call <vilib>:"Read Holding Registers.vi"("error in (no error)"=w387, "quantity"=u16 6 ("number of holding registers"), "starting address"=u16 3840, "MB session in"=w386) -> ("error out"=w374:errorcluster, "Registers"=w390:u16[], "MB session out"=w404:refnum<class "MB_Master.lvclass">)  [unwired: 5 in]
            n243 = case shown="无错误" w374 {
              tunnel: w390 -> [w419 _]
              frame No Error {
                n244 = Array To Cluster(array=w419) -> (cluster=w420:T36)
                n245 = To Word Integer(number=w419) -> (16bit integer=w418:i16[])
                n246 = global write "采配水全局变量.vi" "AD"(w420) -> ()
                n247 = formula code="float AD0,AD1,AD2,AD3,AD4,AD5,AD6;\n\nAD0 = IN[0]*0.0213643-74.9947;\nAD1 = IN[1]*0.0152602-24.9962;\nAD2 = (IN[2]/65.53-25)/100;\nAD3 = (IN[3]/65.53-25)/100;\nAD4 = IN[4];\nAD5 = IN[5];"("IN"=w418) -> ("AD0"=w417:dbl, "AD1"=w416:dbl, "AD2"=w412:dbl, "AD3"=w411:dbl, "AD4"=w415:dbl, "AD5"=w414:dbl)
                "过滤压力" <- w412
                "供水压力" <- w411
                n248 = Bundle(w417, w416, w412, w411, w415, w414) -> (w413:cluster{dbl, dbl, dbl, dbl, dbl, dbl})  [unwired: 1 in]
                n249 = global write "采配水全局变量.vi" "转换值"(w413) -> ()
              }
              frame Error {
              }
            }
            n250 = call <vilib>:"Read Coils.vi"("error in (no error)"=w374, "quantity"=u16 34 ("number of coils"), "starting address"=u16 0, "MB session in"=w404) -> ("error out"=w400:errorcluster, "Coils"=w391:bool[], "MB session out"=w401:refnum<class "MB_Master.lvclass">)  [unwired: 5 in]
            n251 = global write "采配水全局变量.vi" "输出状态"(w391) -> ()
            n252 = call <vilib>:"Read Coils.vi"("error in (no error)"=w400, "quantity"=u16 16 ("number of coils"), "starting address"=u16 1000, "MB session in"=w401) -> ("error out"=w396:errorcluster, "Coils"=w392:bool[], "MB session out"=w397:refnum<class "MB_Master.lvclass">)  [unwired: 5 in]
            n253 = global write "采配水全局变量.vi" "输入状态"(w392) -> ()
            n254 = call <vilib>:"Read Coils.vi"("error in (no error)"=w396, "quantity"=u16 16 ("number of coils"), "starting address"=u16 2500, "MB session in"=w397) -> ("error out"=w381:errorcluster, "Coils"=w393:bool[], "MB session out"=w383:refnum<class "MB_Master.lvclass">)  [unwired: 5 in]
            n255 = global write "采配水全局变量.vi" "报警簇"(w393) -> ()
            n256 = call <vilib>:"Read Coils.vi"("error in (no error)"=w381, "quantity"=u16 2 ("starting address"), "starting address"=u16 2802, "MB session in"=w383) -> ("error out"=w378:errorcluster, "Coils"=w377:bool[], "MB session out"=w382:refnum<class "MB_Master.lvclass">)  [unwired: 5 in]
            n257 = Index Array(array=w377) -> (element #1=w376:bool, element #2=w373:bool)  [unwired: 2 in]
            n258 = local write "三级过滤系统"(w376) -> ()
            n259 = local write "63μm反冲洗阀启用"(w373) -> ()
          }
          frame "读参数" {
            n260 = call <vilib>:"Read Holding Registers.vi"("error in (no error)"=w433, "quantity"=u16 37 ("number of holding registers"), "starting address"=u16 100, "MB session in"=w434) -> ("error out"=w428:errorcluster, "Registers"=w430:u16[], "MB session out"=w429:refnum<class "MB_Master.lvclass">)  [unwired: 5 in]
            n261 = Array To Cluster(array=w430) -> (cluster=w427:T37)
            n262 = global write "采配水全局变量.vi" "参数设置"(w427) -> ()
          }
          frame "多个写入" {
            n263 = Unbundle By Name(w440) -> ("数据"=w439:variant)
            n264 = Variant To Data(type=T31 {"starting address"=0, "holding register values"=[]}, Variant=w439) -> (data=w437:T31)  [unwired: 1 in, 1 out]
            n265 = Unbundle By Name(w437) -> ("starting address"=w436:u16, "holding register values"=w435:u16[])
            n266 = call <vilib>:"Write Multiple Registers.vi"("error in (no error)"=w443, "values"=w435, "starting address"=w436, "MB session in"=w444) -> ("error out"=w442:errorcluster, "MB session out"=w441:refnum<class "MB_Master.lvclass">)  [unwired: 6 in]
          }
          frame "单个写入" {
            n267 = Unbundle By Name(w450) -> ("数据"=w449:variant)
            n268 = Variant To Data(type=T32 {"starting address"=0, "holding register value"=0}, Variant=w449) -> (data=w447:T32)  [unwired: 1 in, 1 out]
            n269 = Unbundle By Name(w447) -> ("starting address"=w446:u16, "holding register value"=w445:u16)
            n270 = call <vilib>:"Write Single Register.vi"("error in (no error)"=w453, "value"=w445, "address"=w446, "MB session in"=w454) -> ("error out"=w452:errorcluster, "MB session out"=w451:refnum<class "MB_Master.lvclass">)  [unwired: 6 in]
          }
          frame "线圈写入" {
            n271 = Unbundle By Name(w460) -> ("数据"=w459:variant)
            n272 = Variant To Data(type=T33 {"starting address"=0, "coil values"=[]}, Variant=w459) -> (data=w457:T33)  [unwired: 1 in, 1 out]
            n273 = Unbundle By Name(w457) -> ("starting address"=w456:u16, "coil values"=w455:bool[])
            n274 = call <vilib>:"Write Multiple Coils.vi"("error in (no error)"=w463, "values"=w455, "starting address"=w456, "MB session in"=w464) -> ("error out"=w462:errorcluster, "MB session out"=w461:refnum<class "MB_Master.lvclass">)  [unwired: 6 in]
          }
          frame "shutdown" {
            n275 = call <vilib>:"Write Single Register.vi"("error in (no error)"=w468, "value"=u16 0, "address"=u16 4047, "MB session in"=w472) -> ("error out"=w467:errorcluster, "MB session out"=w471:refnum<class "MB_Master.lvclass">)  [unwired: 6 in]
            n276 = call-dynamic "Close Session.vi"("error in (no error)"=w467, "MB session in"=w471) -> ("error out"=w473:errorcluster)  [unwired: 9 in]
            n277 = call <vilib>:"Clear Errors.vi"("error in (no error)"=w473) -> ("error out"=w466:errorcluster)  [unwired: 5 in, 1 out]
            n278 = call "调用WinProladder.vi"("错误输入（无错误）"=w466) -> ("错误输出"=w465:errorcluster)  [unwired: 10 in]
          }
        }
        n279 = Unbundle By Name(w326) -> ("status"=w325:bool)
      }
      frame Error {
        n280 = property class="MB_Master"(reference=w477) -> (reference out=w476:refnum<class "MB_Master.lvclass">, "Properties:Session Valid"=w478:bool)  [unwired: 1 in, 1 out]
        n281 = Flush Queue(queue=w483) -> (queue out=w482:refnum<queue>)  [unwired: 1 in, 2 out]
        n282 = Wait (ms)(milliseconds to wait=u32 2000 ("等待时间（毫秒）")) -> ()  [unwired: 1 out]
        n283 = case shown="假" w478 {
          tunnel: w482 -> [w485 _]
          frame False {
            n284 = Enqueue Element At Opposite End(queue=w485, element=cluster{"命令":string, "数据":variant} {"命令"="init", "数据"=variant} ("元素")) -> ()  [unwired: 2 in, 3 out]
          }
          frame True {
          }
        }
        n285 = call <vilib>:"Clear Errors.vi"("error in (no error)"=w479) -> ("error out"=w480:errorcluster)  [unwired: 5 in, 1 out]
      }
    }
    "通讯故障" <- w317
    n286 = global write "采配水全局变量.vi" "通讯故障"(w317) -> ()
  }
  n287 = call-dynamic "Close Session.vi"("error in (no error)"=w4, "MB session in"=w6) -> ()  [unwired: 9 in, 1 out]
